vi "Measure_SubArray(SubVI).vi"(8 "error in (no error)":errorcluster, 9 "FinalPos":dbl, 10 "StartPos":dbl, 11 "InArray":dbl[](array[numeric])) -> (0 "error out":errorcluster, 2 "Output cluster":cluster{dbl, dbl, "Numeric Control":dbl}, 3 "OutSubArray":dbl[](array[numeric]))   [LabVIEW 2014]
doc: "This SubVI calculate SubArray based on start and finish position graph cursors. Then it measure START. MAX and MIN in this SubArray"
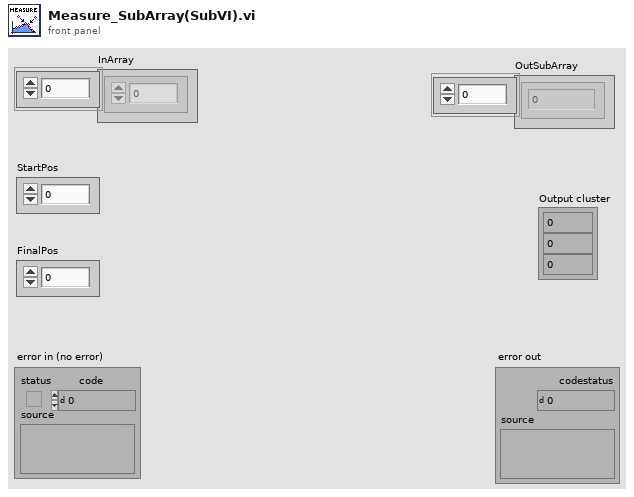
[diagram p1: front panel]
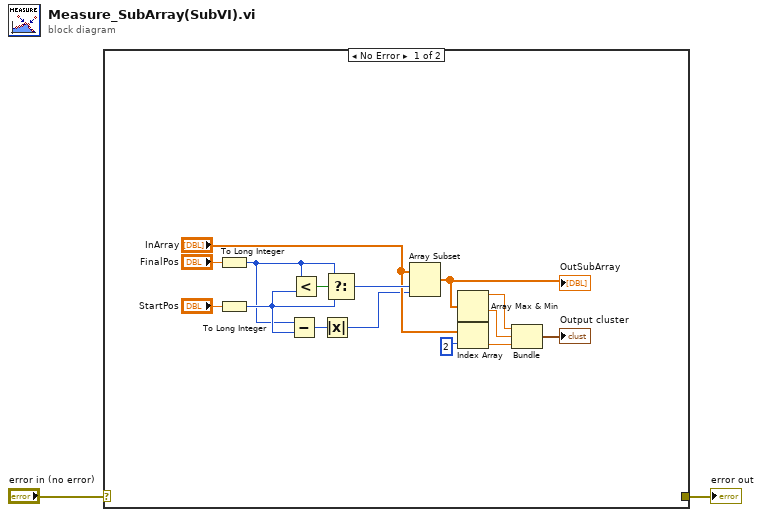
[diagram p0: block diagram]
diagram:
  n1 = case shown="No Error" "error in (no error)" {
    selector: "error in (no error)" -> [_ w18]
    tunnel: [_ w18] -> w1
    frame No Error {
      n2 = To Long Integer(number="FinalPos") -> (32bit integer=w13:i32)
      n3 = To Long Integer(number="StartPos") -> (32bit integer=w14:i32)
      n4 = Subtract(x=w13, y=w14) -> (x-y=w8:i32)
      n5 = Less?(x=w13, y=w14) -> (x < y?=w7:bool)
      n6 = Absolute Value(x=w8) -> (abs(x)=w9:i32)
      n7 = Select(t=w13, s=w7, f=w14) -> (s? t:f=w15:i32)
      n8 = Array Subset(array="InArray", index=w15, length=w9) -> (w16:dbl[])
      "OutSubArray" <- w16
      n9 = Array Max & Min(array=w16) -> (max value=w4:dbl, min value=w5:dbl)  [unwired: 2 out]
      n10 = Index Array(array="InArray", index=2) -> (element=w6:dbl)
      n11 = Bundle(w4, w5, "Numeric Control"=w6) -> (→"Output cluster":cluster{dbl, dbl, "Numeric Control":dbl})  [unwired: 1 in]
    }
    frame Error {
    }
  }
  "error out" <- w1
